vi "Acquire DeviceComms.vi"(8 "error in (no error)":errorcluster, 9 "Timeout ms (1000)":i32=1000, 11 "Session in":refnum<class "Session.lvclass">) -> (0 "error out":errorcluster, 2 "DeviceComms":refnum<class "DeviceComms.lvclass">, 3 "Session out":refnum<class "Session.lvclass">)   [LabVIEW 2024, in "CTI.lvlib" / "Session.lvclass"]
doc: "Acquires the DeviceComm instance that is used to interact with a device. This VI can be used by connection wrapper classes and peripheral classes to safely perform a handful of device operations without being interrupted by other parallel loops. Be sure to return the DeviceComms instance by calling <b>Return DeviceComms.vi</b> otherwise the session will fail to perform as expected and future attempts to interact with the device will fail."
uses:
  Session.lvclass
  DeviceComms/DeviceComms.lvclass
  Session.lvclass/Session.ctl
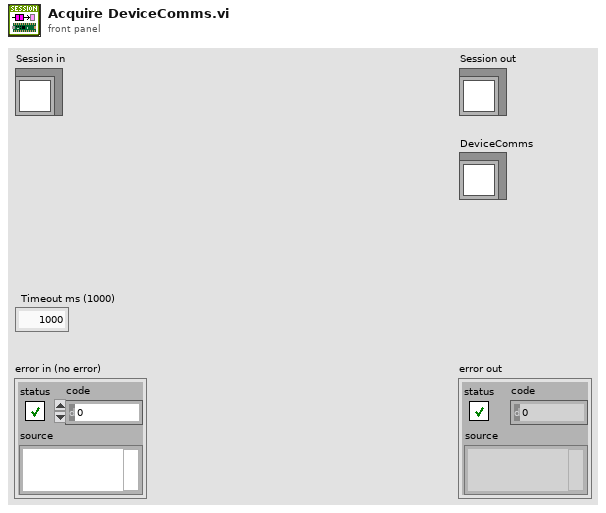
[diagram p1: front panel]
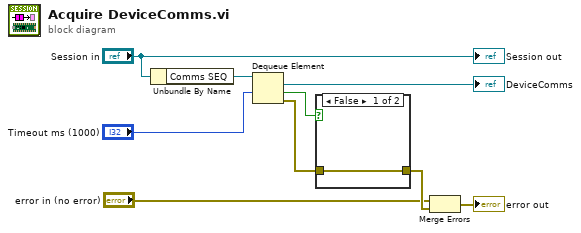
[diagram p0: block diagram]
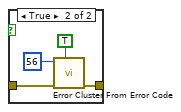
[diagram p2: hidden frame]
diagram:
  n1 = Unbundle By Name("Session in") -> ("Comms SEQ"=w8:refnum<queue>)
  n2 = Dequeue Element(queue=w8, timeout in ms (-1)="Timeout ms (1000)") -> (element=→"DeviceComms":refnum<class "DeviceComms.lvclass">, timed out?=w5:bool, error out=w4:errorcluster)  [unwired: 1 in, 1 out]
  n3 = case shown="False" w5 {
    tunnel: w4 -> [w10 w14]
    tunnel: [w10 w11] -> w3
    frame False {
    }
    frame True {
      n4 = call <vilib>:"Error Cluster From Error Code.vi"("show call chain? (False)"=TRUE, "error in (no error)"=w14, "error code (0)"=56) -> ("error out"=w11:errorcluster)  [unwired: 6 in]
    }
  }
  n5 = Merge Errors("error in (no error)", w3) -> (→"error out":errorcluster)
  "Session out" <- "Session in"
